vi "Create Target Listener.vi"(8 "error in":errorcluster) -> (0 "error out":errorcluster, 3 "Queue out":refnum<queue>)   [LabVIEW 2016, in "Vision Server.lvclass"]
uses:
  Vision Server.lvclass
  typedef/Target Message JSON.ctl
  typedef/Target Vector.ctl
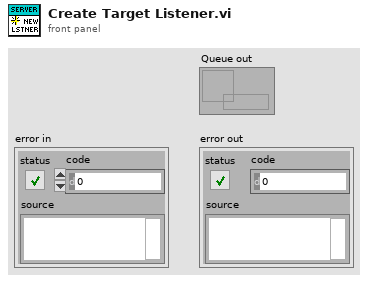
[diagram p1: front panel]
types:
  T1 = typedef "Vision Server.lvclass/Target Message JSON.ctl" = cluster{"capturedAgoMs":i32, "targets":T2[]}
  T2 = typedef "Vision Server.lvclass/Target Vector.ctl" = cluster{"y":dbl, "z":dbl}
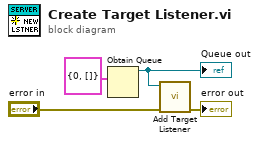
[diagram p0: block diagram]
diagram:
  n1 = Obtain Queue(element data type=T1 {"capturedAgoMs"=0, "targets"=[]} ("Target Msg")) -> (queue out=w3:refnum<queue>)  [unwired: 4 in, 2 out]
  "Queue out" <- w3
  n2 = call "Add Target Listener.vi"("error in"="error in", "queue out"=w3) -> ("error out"=→"error out":errorcluster)  [unwired: 9 in]
